vi "_DRIVER_SHARED_INI_Create-Default-File.vi"(8 "error in (no error)":errorcluster, 11 "How many Boards?":i32) -> (0 "error out":errorcluster, 3 "path":path)   [LabVIEW 2020]
doc: "Generate the default \"_HW-Configuration_.ini\" in %temp%"
uses:
  TYPEDEF/_DRIVER_SHARED_TYPEDEF_INI-Method.ctl
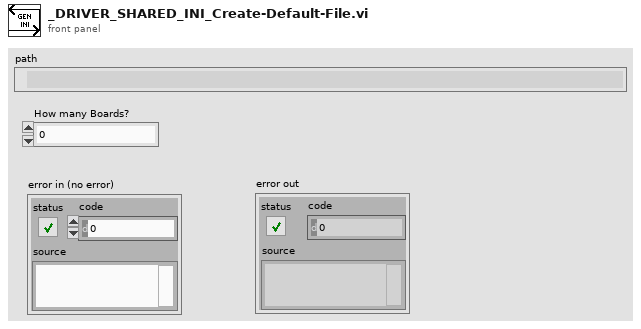
[diagram p1: front panel]
types:
  T1 = typedef "_DRIVER_SHARED_TYPEDEF_INI-Method.ctl" = enum16{"OPEN/CREATE", "READ", "WRITE", "CLOSE", "NO_OP"}
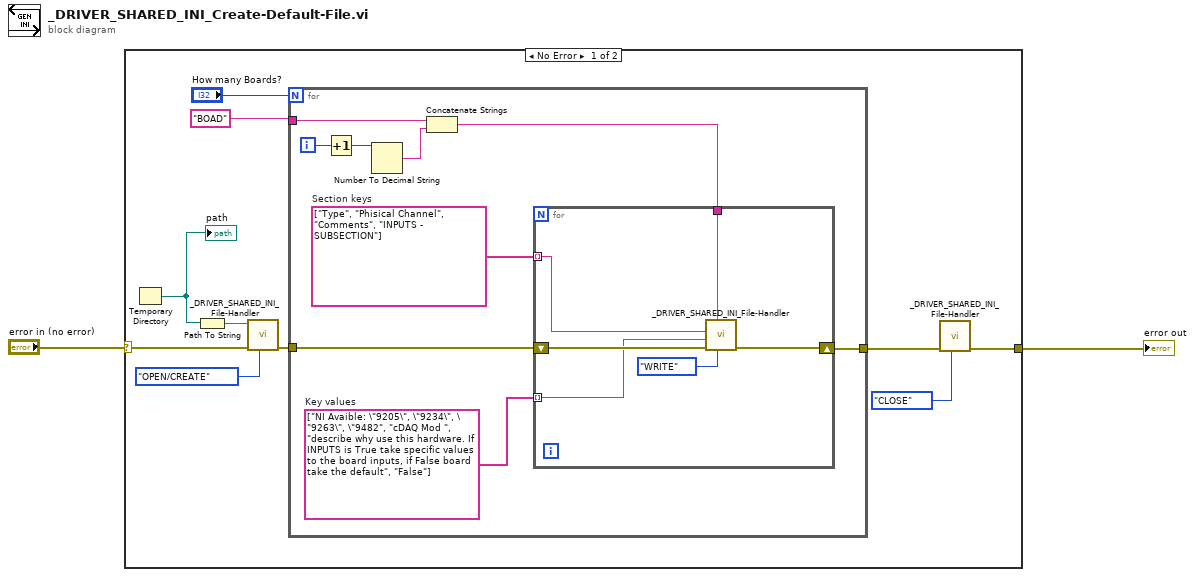
[diagram p0: block diagram]
diagram:
  n1 = case shown="No Error" "error in (no error)" {
    selector: "error in (no error)" -> [w6 w28]
    tunnel: [w3 w28] -> w1
    frame No Error {
      n2 = Temporary Directory() -> (w11:path)
      "path" <- w11
      n3 = Path To String(path=w11) -> (string=w10:string)
      n4 = call "_DRIVER_SHARED_INI_File-Handler.vi"("INI-FileMethod"=_DRIVER_SHARED_TYPEDEF_INI-Method."OPEN/CREATE", "error in (no error)"=w6, "Path File"=w10) -> ("error out"=w9:errorcluster)  [unwired: 6 in, 2 out]
      n5 = for {
        N: "How many Boards?" -> [_]
        tunnel: w9 -> [w21]
        tunnel: "BOAD" ("section IN") -> [w17]
        tunnel: [w14] -> w4
        i -> [w18]
        w19 = string[] ["NI Avaible: \"9205\", \"9234\", \"9263\", \"9482", "cDAQ Mod ", "describe why use this hardware. If INPUTS is True take specific values to the board inputs, if False board take the default", "False"]  # Key values
        w20 = string[] ["Type", "Phisical Channel", "Comments", "INPUTS - SUBSECTION"]  # Section keys
        n6 = Increment(x=w18) -> (x+1=w13:i32)
        n7 = Number To Decimal String(number=w13) -> (decimal integer string=w16:string)  [unwired: 1 in]
        n8 = Concatenate Strings(w17, w16) -> (w15:string)
        n9 = for {
          tunnel: w20 -> [w24] mode=indexing
          tunnel: w19 -> [w23] mode=indexing
          tunnel: w15 -> [w26]
          shift-right: [w22] -> w14
          shift-left: w21 -> [w25]
          n10 = call "_DRIVER_SHARED_INI_File-Handler.vi"("INI-FileMethod"=_DRIVER_SHARED_TYPEDEF_INI-Method."WRITE", "section IN"=w26, "error in (no error)"=w25, "Value to write"=w23, "key IN"=w24) -> ("error out"=w22:errorcluster)  [unwired: 4 in, 2 out]
        }
      }
      n11 = call "_DRIVER_SHARED_INI_File-Handler.vi"("INI-FileMethod"=_DRIVER_SHARED_TYPEDEF_INI-Method."CLOSE", "error in (no error)"=w4) -> ("error out"=w3:errorcluster)  [unwired: 7 in, 2 out]
    }
    frame Error {
    }
  }
  "error out" <- w1
